vi "Make Value String.vi"(5 "Initial String (\"\")":string, 7 "Int Value (0)":i32, 9 "Float Value (0)":dbl, 11 "Error In":errorcluster caption="エラー入力", 12 "Kind Of Value (0: Int)":i32(ring) items=["Int", "Float"], 13 "Float Decimal Position (1)":i32=1) -> (6 "Resulting String":string, 15 "Error Out":errorcluster caption="エラー出力")   [LabVIEW 2020, in "Yokogawa GX Series.lvlib"]
doc: "Adds quote to string and concatenate to initial string."
uses:
  <instrlib>/Yokogawa GX Series/Yokogawa GX Series.lvlib
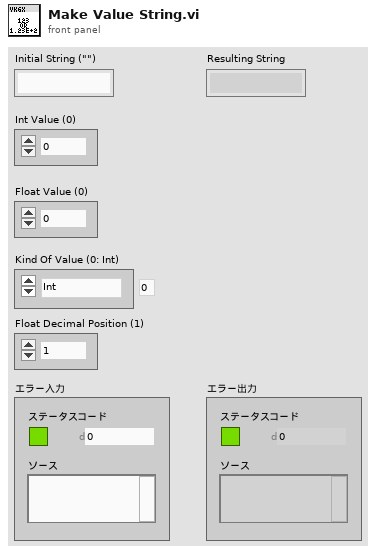
[diagram p1: front panel]
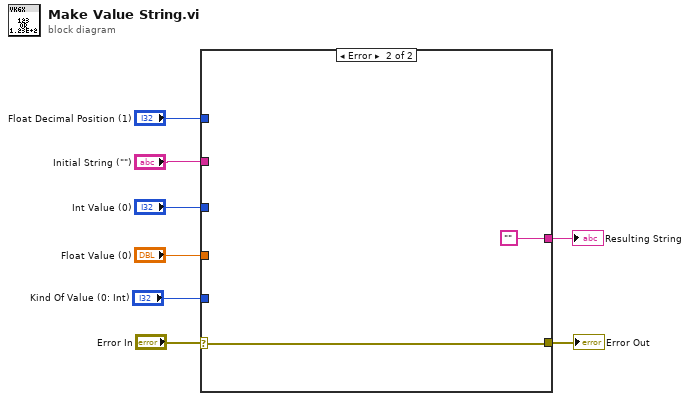
[diagram p0: block diagram]
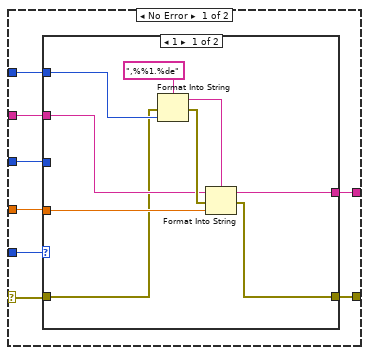
[diagram p2: hidden frame]
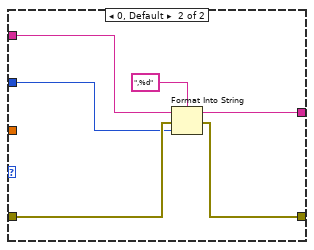
[diagram p3: hidden frame]
diagram:
  n1 = case shown="Error" "Error In" {
    selector: "Error In" -> [w9 w33]
    tunnel: "Initial String (\"\")" -> [w16 _]
    tunnel: "Int Value (0)" -> [w15 _]
    tunnel: "Float Value (0)" -> [w14 _]
    tunnel: "Float Decimal Position (1)" -> [w13 _]
    tunnel: [w12 w33] -> w4
    tunnel: [w11 ""] -> w3
    tunnel: "Kind Of Value (0: Int)" -> [w10 _]
    frame No Error {
      n2 = case shown="1" w10 {
        tunnel: w9 -> [w19 w27]
        tunnel: w16 -> [w21 w31]
        tunnel: w15 -> [_ w26]
        tunnel: w14 -> [w20 _]
        tunnel: w13 -> [w22 _]
        tunnel: [w18 w30] -> w12
        tunnel: [w17 w29] -> w11
        frame 1 {
          n3 = Format Into String(format string=",%%1.%de", error in=w19, w22) -> (resulting string=w23:string, error out=w24:errorcluster)  [unwired: 1 in]
          n4 = Format Into String(format string=w23, initial string=w21, error in=w24, w20) -> (resulting string=w17:string, error out=w18:errorcluster)
        }
        frame 0, Default {
          n5 = Format Into String(format string=",%d", initial string=w31, error in=w27, w26) -> (resulting string=w29:string, error out=w30:errorcluster)
        }
      }
    }
    frame Error {
    }
  }
  "Resulting String" <- w3
  "Error Out" <- w4
